vi "CasesOfTheSteps.vi"(0 "GEA2 Reference In":refnum<k24>, 5 "session in":refnum<k35>, 7 "Cluster":T2) -> (4 "GEA2 Reference Out":refnum<k24>, 6 "session out":refnum<k35>, 8 "Results":T1)   [LabVIEW 2023]
uses:
  D:/Common/LabVIEW GEA2 Toolkit/source/GEA3 DLL Source/GeaCommunication.dll
  Common/LabVIEW GEA2 Toolkit/source/GEA3 DLL Source/GeaCommunication.dll
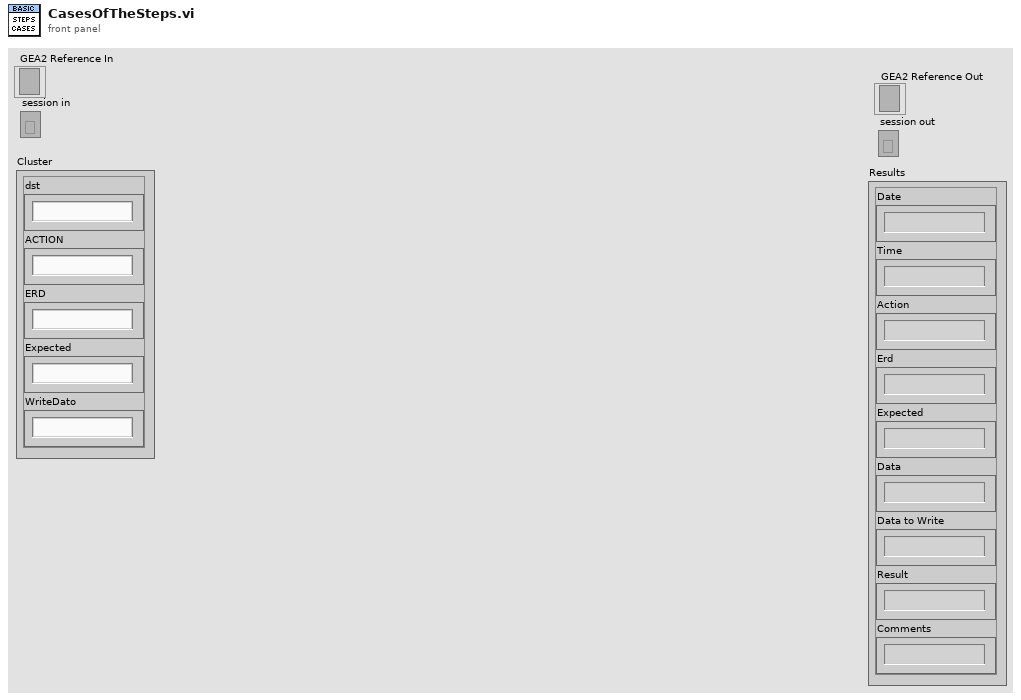
[diagram p1: front panel]
types:
  T1 = cluster{"Date":string, "Time":string, "Action":string, "Erd":string, "Expected":string, "Data":string, "Data to Write":string, "Result":string, "Comments":string}
  T2 = cluster{"dst":string, "ACTION":string, "ERD":string, "Expected":string, "WriteDato":string}
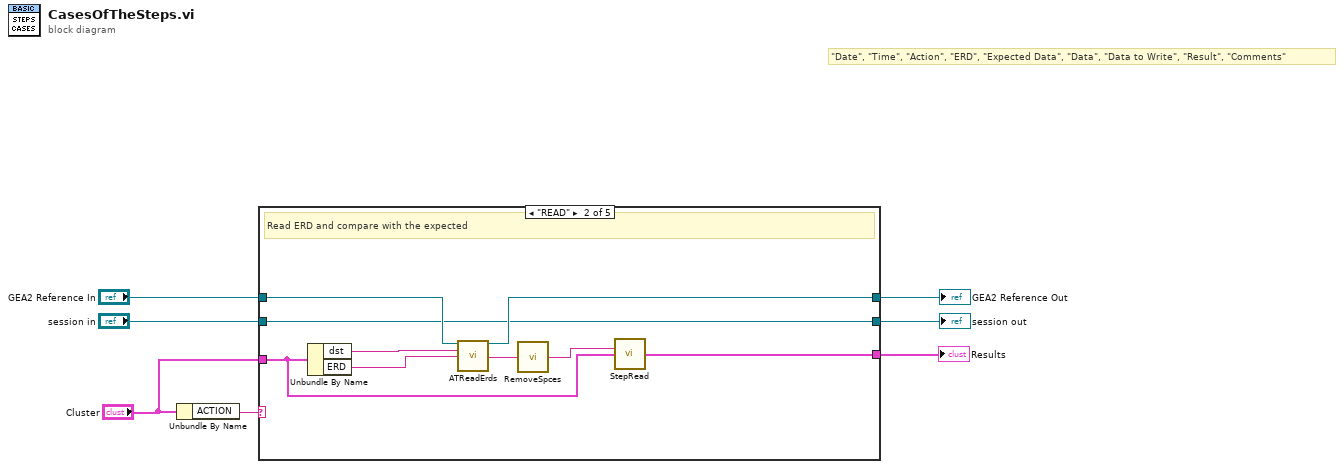
[diagram p0: block diagram]
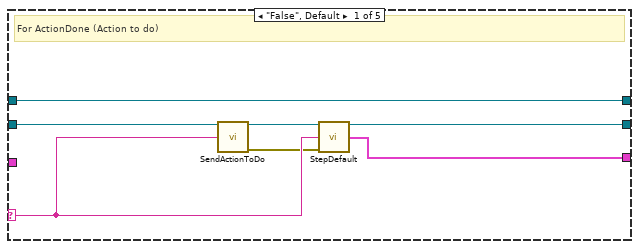
[diagram p2: hidden frame]
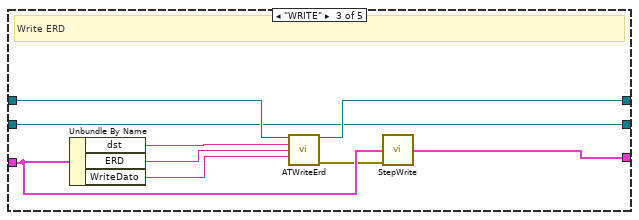
[diagram p3: hidden frame]
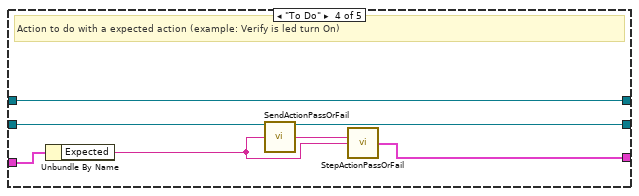
[diagram p4: hidden frame]
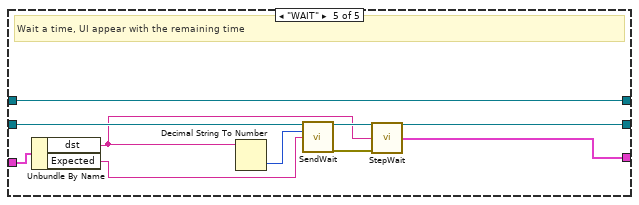
[diagram p5: hidden frame]
diagram:
  # "\"Date\", \"Time\", \"Action\", \"ERD\", \"Expected Data\", \"Data\", \"Data to Write\", \"Result\", \"Comments\""
  n1 = Unbundle By Name("Cluster") -> ("ACTION"=w7:string)
  n2 = case shown="\"READ\"" w7 {
    selector: w7 -> [w10 _ _ _ _]
    tunnel: [w13 w22 w31 w36 w43] -> w2
    tunnel: [w11 w20 w29 w38 w47] -> w1
    tunnel: "GEA2 Reference In" -> [w13 w21 w30 w36 w43]
    tunnel: "session in" -> [w12 w20 w29 w37 w45]
    tunnel: "Cluster" -> [_ w15 w25 w35 w44]
    tunnel: [w8 w14 w24 w32 w40] -> w3
    frame "False", Default {
      # "For ActionDone (Action to do)"
      n3 = call "SendActionToDo.vi"("session in"=w12, "Action ToDo"=w10) -> ("session out"=w11:refnum<k35>, "error out"=w9:errorcluster)  [unwired: 12 in]
      n4 = call "StepDefault.vi"("Action"=w10, "error in"=w9) -> ("Results"=w8:T1)  [unwired: 12 in, 1 out]
    }
    frame "READ" {
      # "Read ERD and compare with the expected"
      n5 = Unbundle By Name(w15) -> ("dst"=w19:string, "ERD"=w18:string)
      n6 = call "ATReadErds.vi"("GEA2 Reference In"=w21, "Destination"=w19, "Erd Number"=w18) -> ("GEA2 Reference Out"=w22:refnum<k24>, "ERD Data Out"=w17:string)  [unwired: 10 in, 1 out]
      n7 = call "RemoveSpces.vi"("input string"=w17) -> ("result string"=w16:string)  [unwired: 14 in]
      n8 = call "StepRead.vi"("Data Read"=w16, "Cluster in"=w15) -> ("Results"=w14:T1)  [unwired: 13 in]
    }
    frame "WRITE" {
      # "Write ERD"
      n9 = Unbundle By Name(w25) -> ("dst"=w28:string, "ERD"=w27:string, "WriteDato"=w26:string)
      n10 = call "ATWriteErd.vi"("GEA2 Reference In"=w30, "Destination"=w28, "Erd Number"=w27, "Data to write"=w26) -> ("GEA2 Reference Out"=w31:refnum<k24>, "Error Out"=w23:errorcluster)  [unwired: 10 in]
      n11 = call "StepWrite.vi"("Cluster in"=w25, "error in"=w23) -> ("Results"=w24:T1)  [unwired: 12 in, 1 out]
    }
    frame "To Do" {
      # "Action to do with a expected action (example: Verify is led turn On)"
      n12 = Unbundle By Name(w35) -> ("Expected"=w33:string)
      n13 = call "SendActionPassOrFail.vi"("session in"=w37, "Action ToDo"=w33) -> ("session out"=w38:refnum<k35>, "Pass or Fail"=w34:string)  [unwired: 11 in, 1 out]
      n14 = call "StepActionPassOrFail.vi"("Result"=w34, "Expected"=w33) -> ("Results"=w32:T1)  [unwired: 13 in]
    }
    frame "WAIT" {
      # "Wait a time, UI appear with the remaining time"
      n15 = Unbundle By Name(w44) -> ("dst"=w41:string, "Expected"=w42:string)
      n16 = Decimal String To Number(string=w41) -> (number=w46:i32)  [unwired: 2 in, 1 out]
      n17 = call "SendWait.vi"("session in"=w45, "Time (s)"=w46, "Text To Wait"=w42) -> ("session out"=w47:refnum<k35>, "error out"=w39:errorcluster)  [unwired: 11 in]
      n18 = call "StepWait.vi"("Time to wait"=w41, "error in"=w39) -> ("Results"=w40:T1)  [unwired: 12 in, 1 out]
    }
  }
  "Results" <- w3
  "GEA2 Reference Out" <- w2
  "session out" <- w1
